vi "instanciateHtmlConverter.vi"(8 "error in (no error)":errorcluster, 11 "workbook":refnum<k24>) -> (0 "error out":errorcluster, 3 "ExcelToHtmlConverter":refnum<k24>)   [LabVIEW 2017, in "LabVIEW NPOI.lvlib" / "MS-Excel.lvclass"]
uses:
  MS-Excel.lvclass
  C:/Users/Neo/Desktop/Dev_Tools_BR/LabVIEW_NPOI/src/lib/NPOI 2.1.1/NPOI.dll
  lib/NPOI 2.1.1/NPOI.dll
  C:/Users/Neo/Desktop/Dev_Tools_BR/LabVIEW_NPOI/src/lib/NPOI 2.1.1/NPOI.OOXML.dll
  lib/NPOI 2.1.1/NPOI.OOXML.dll
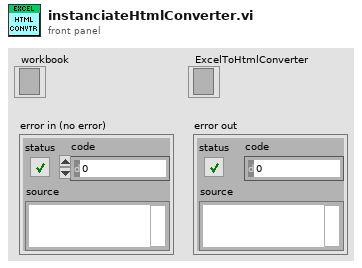
[diagram p1: front panel]
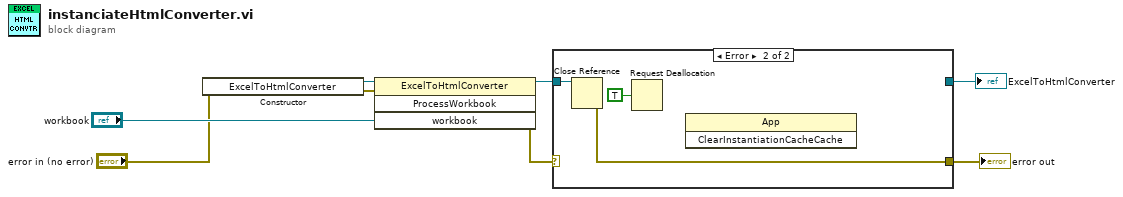
[diagram p0: block diagram]
diagram:
  n1 = constructor class="ExcelToHtmlConverter"(error in="error in (no error)") -> (reference out=w8:refnum<k24>, error out=w7:errorcluster)  [unwired: 2 in, 1 out]
  n2 = invoke class="ExcelToHtmlConverter" method="ProcessWorkbook"(reference=w8, error in=w7, "workbook"="workbook") -> (reference out=w6:refnum<k24>, error out=w5:errorcluster)  [unwired: 1 in, 2 out]
  n3 = case shown="Error" w5 {
    selector: w5 -> [w10 _]
    tunnel: [w10 w12] -> w2
    tunnel: w6 -> [w9 w13]
    tunnel: [w9 _] -> w1
    frame No Error {
    }
    frame Error {
      n4 = Close Reference(reference=w13) -> (error out=w12:errorcluster)  [unwired: 1 in]
      n5 = Request Deallocation(TRUE ("flag")) -> ()
      n6 = invoke class="App" method="ClearInstantiationCacheCache"() -> ()  [unwired: 3 in, 3 out]
    }
  }
  "error out" <- w2
  "ExcelToHtmlConverter" <- w1
